vi "Create.vi"(7 "mode settings":variant, 8 "error in":errorcluster, 9 "number of default channels":i32, 10 "channel settings":variant, 11 "counter driven output mode in":refnum<class "Counter Driven Output Mode.lvclass">) -> (0 "error out":errorcluster, 1 "channels":refnum<class "Channel.lvclass">[](array[class]), 3 "counter driven output mode out":refnum<class "Counter Driven Output Mode.lvclass">)   [LabVIEW 2020, in "Scan Engine Scripting.lvlib" / "Counter Driven Output Mode.lvclass"]
uses:
  Counter Driven Output Mode.lvclass
  Channel Classes/Channel/Channel.lvclass
  Drive from Slot.ctl
  Controls/counter driven output channel settings.ctl
  Channel Classes/Counter Driven Output Channel/Counter Driven State.ctl
  c1346d1a-9a60-41c0-bcc7-db98e9148e52.vi
  Channel Classes/Counter Driven Output Channel/Counter Driven Output Channel.lvclass
  C:/jenkins/workspace/ercat-custom-device_release_20.4/Custom Device Source/Scripting/Modules/Channel Classes/Channel/Channel.lvclass
  Scan Engine Scripting.lvlib
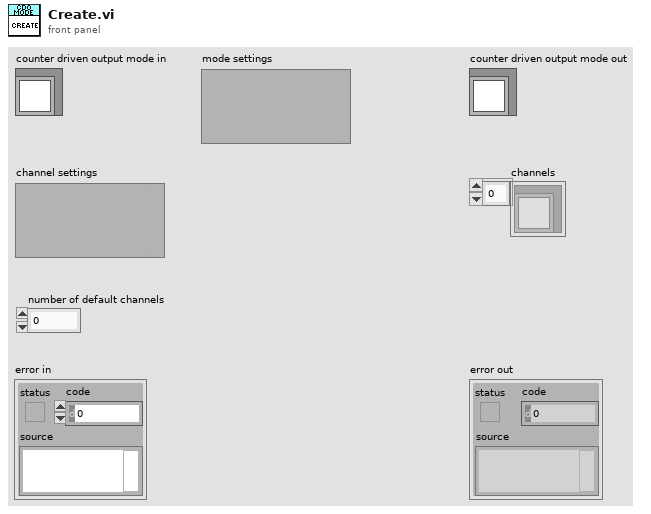
[diagram p1: front panel]
types:
  T1 = typedef "Scan Engine Scripting.lvlib/counter driven output channel settings.ctl" = cluster{"name":string, "default value":bool, "counter driven state":T2}
  T2 = typedef "Scan Engine Scripting.lvlib/Counter Driven Output Channel.lvclass/Counter Driven State.ctl" = enum16{"Disabled", "Enabled"}
  T3 = typedef "Scan Engine Scripting.lvlib/Counter Driven Output Mode.lvclass/Drive from Slot.ctl" = enum16{"Slot 1", "Slot 2", "Slot 3", "Slot 4", "Slot 5", "Slot 6", "Slot 7", "Slot 8"}
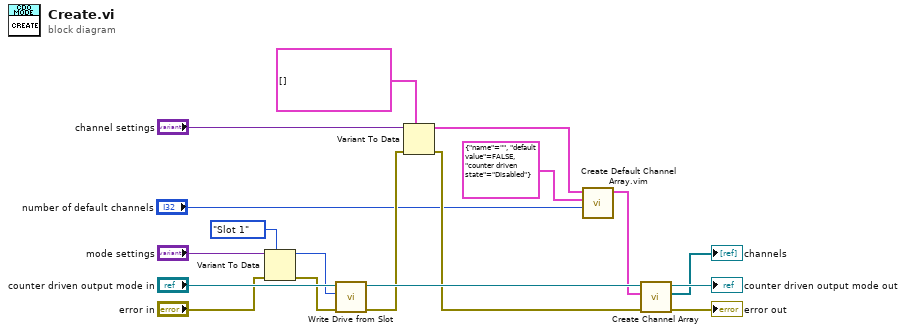
[diagram p0: block diagram]
diagram:
  n1 = Variant To Data(error in="error in", type=Drive_from_Slot."Slot 1" ("mode settings"), Variant="mode settings") -> (data=w12:T3, error out=w11:errorcluster)
  n2 = call-dynamic "Write Drive from Slot.vi"("error in"=w11, "drive from slot"=w12, "counter driven output mode in"="counter driven output mode in") -> ("error out"=w7:errorcluster, "counter driven output mode out"=w18:refnum<class "Counter Driven Output Mode.lvclass">)  [unwired: 7 in]
  n3 = Variant To Data(error in=w7, type=T1[] [] ("channel settings"), Variant="channel settings") -> (data=w3:T1[], error out=w6:errorcluster)
  n4 = call "Create Default Channel Array.vim"("number of default channels"="number of default channels", "default settings"=T1 {"name"="", "default value"=FALSE, "counter driven state"=enum."Disabled"} ("channel settings"), "channel settings in"=w3) -> ("channel settings out"=w2:T1[])  [unwired: 8 in]
  n5 = call "Create Channel Array.vi"("error in"=w6, "channel settings"=w2, "counter driven output mode in"=w18) -> ("error out"=→"error out":errorcluster, "channels"=→"channels":refnum<class "Counter Driven Output Channel.lvclass">[], "counter driven output mode out"=→"counter driven output mode out":refnum<class "Counter Driven Output Mode.lvclass">)  [unwired: 6 in]
